vi "VI Tree - md5__ogtk.vi"   [LabVIEW 2017]
uses:
  <userlib>/_OpenG.lib/md5/md5.llb/MD5 Message Digest (Binary String)__ogtk.vi
panel:
  # "Please visit http://www.OpenG.org to learn about the\nOpen Source LabVIEW software movement.\n\nNOTICE -- YOU MUST LEAVE THIS NOTICE IN PLACE.  PER THE TERMS OF THE LICENSE BELOW, YOU MAY SUBLICENSE THIS SOFTWARE \nIN ANY WAY THAT DOES NOT CONFLICT WITH THIS LICENSE.\n\n### BSD License (http://www.opensource.org/licenses/bsd-license.php) Begin ###\n \nCopyright (c) 2004, Enrique Vargas <vargas@visecurity.com>\n\nAll rights reserved.\n\nRedistribution and use in source and binary forms, with or without modification, are permitted provided that the following conditions are met:\n\n    * Redistributions of source code must retain the above copyright notice, this list of conditions and the following disclaimer.\n    * Redistributions in binary form must reproduce the above copyright notice, this list of conditions and the following disclaimer in the \n       documentation and/or other materials provided with the distribution.\n    * Neither the name of SciWare, James Kring, Inc., nor the names of its contributors may be used to endorse or promote products derived \n       from this software without specific prior written permission.\n\nTHIS SOFTWARE IS PROVIDED BY THE COPYRIGHT HOLDERS AND CONTRIBUTORS \"AS IS\" AND ANY EXPRESS OR IMPLIED WARRANTIES, \nINCLUDING, BUT NOT LIMITED TO, THE IMPLIED WARRANTIES OF MERCHANTABILITY AND FITNESS FOR A PARTICULAR PURPOSE ARE \nDISCLAIMED. IN NO EVENT SHALL THE COPYRIGHT OWNER OR CONTRIBUTORS BE LIABLE FOR ANY DIRECT, INDIRECT, INCIDENTAL,\n SPECIAL, EXEMPLARY, OR CONSEQUENTIAL DAMAGES (INCLUDING, BUT NOT LIMITED TO, PROCUREMENT OF SUBSTITUTE GOODS OR \nSERVICES; LOSS OF USE, DATA, OR PROFITS; OR BUSINESS INTERRUPTION) HOWEVER CAUSED AND ON ANY THEORY OF LIABILITY, \nWHETHER IN CONTRACT, STRICT LIABILITY, OR TORT (INCLUDING NEGLIGENCE OR OTHERWISE) ARISING IN ANY WAY OUT OF THE USE \nOF THIS SOFTWARE, EVEN IF ADVISED OF THE POSSIBILITY OF SUCH DAMAGE.\n\n### BSD License End ###"
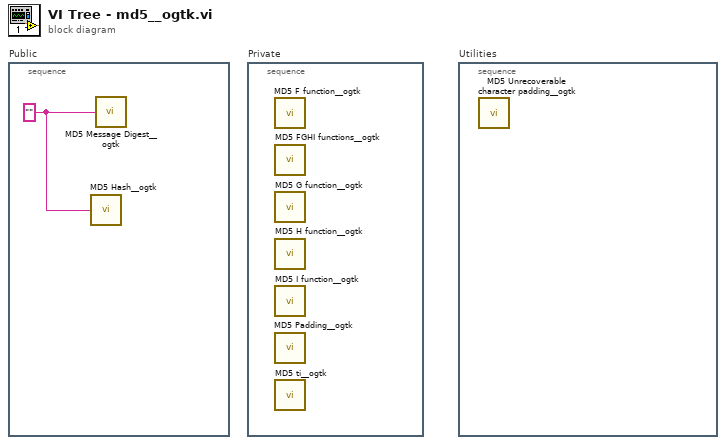
[diagram p0: block diagram]
diagram:
  n1 = stacked-sequence "Public" {
    frame #0 {
      w1 = "" ("Message")
      n2 = call <userlib>:"MD5 Hash__ogtk.vi"("Input String"=w1) -> ()  [unwired: 3 in, 1 out]
      n3 = call-poly <userlib>:"MD5 Message Digest__ogtk.vi"("Message"=w1) -> ()  [unwired: 1 out]
    }
  }
  n4 = stacked-sequence "Private" {
    frame #0 {
      n5 = call <userlib>:"MD5 F function__ogtk.vi"() -> ()  [unwired: 3 in, 1 out]
      n6 = call <userlib>:"MD5 FGHI functions__ogtk.vi"() -> ()  [unwired: 11 in, 1 out]
      n7 = call <userlib>:"MD5 G function__ogtk.vi"() -> ()  [unwired: 3 in, 1 out]
      n8 = call <userlib>:"MD5 H function__ogtk.vi"() -> ()  [unwired: 3 in, 1 out]
      n9 = call <userlib>:"MD5 I function__ogtk.vi"() -> ()  [unwired: 3 in, 1 out]
      n10 = call <userlib>:"MD5 Padding__ogtk.vi"() -> ()  [unwired: 1 in, 1 out]
      n11 = call <userlib>:"MD5 ti__ogtk.vi"() -> ()  [unwired: 1 in, 1 out]
    }
  }
  n12 = stacked-sequence "Utilities" {
    frame #0 {
      n13 = call <userlib>:"MD5 Unrecoverable character padding__ogtk.vi"() -> ()  [unwired: 5 in, 1 out]
    }
  }
